vi "Convert_json_response_to_cluster_response.vi"(11 "Json_Response_in":string) -> (3 "Response":T1)   [LabVIEW 2015]
uses:
  Share Data/uPower_kit.ctl
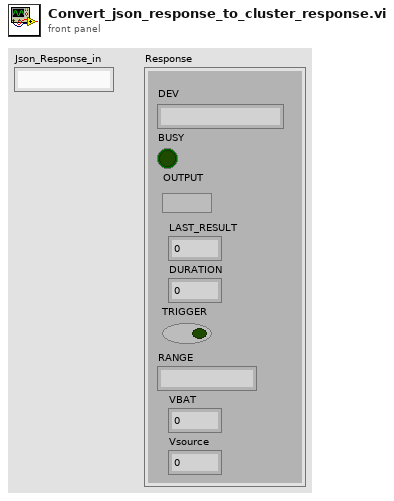
[diagram p1: front panel]
types:
  T1 = typedef "uPower_kit.ctl" = cluster{"DEV":string, "BUSY":bool, "VBAT":dbl, "OUTPUT":bool, "LAST_RESULT":dbl, "DURATION":u16, "TRIGGER":bool, "RANGE":string, "Vsource":dbl}
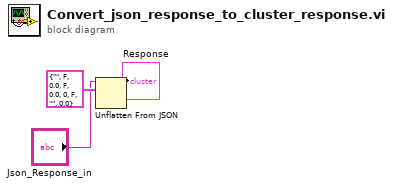
[diagram p0: block diagram]
diagram:
  n1 = Unflatten From JSON(JSON string="Json_Response_in", type and defaults=T1 {"DEV"="", "BUSY"=FALSE, "VBAT"=0.0, "OUTPUT"=FALSE, "LAST_RESULT"=0.0, "DURATION"=0, "TRIGGER"=FALSE, "RANGE"="", "Vsource"=0.0} ("DEV_BUSY")) -> (value=→"Response":T1)  [unwired: 5 in, 1 out]
